vi "dotNETChart_Settings_Default.vi"() -> (2 "Chart Settings clstr":T1={"Enable Mouse Zoom (only works in 2D mode)"=TRUE, "Chart Wall Transparency Level"=37, "Chart Wall Colour"=0, "x axis label"="X axis title", "y axis label"="Y axis title", "Enable3D"=TRUE, "3D Settings"={"Inclination"=20, "LightStyle"=2, "Perspective"=4, "WallWidth"=5, "Rotation"=25}, "BackGradientStyle"=2, "SkinStyle"=1, "Chart Background Gradient Colour"=0, "Chart Border Colour"=0, "Palette"=12, "LegendStyle"=0, "ChartType"=[10, 13], "SeriesDataColour"=[]} {"ChartType" items=["Point", "FastPoint", "Bubble", "Line", "Spline", "StepLine", "FastLine", "Bar", "StackedBar", "StackedBar100", "Column", "StackedColumn", "StackedColumn100", "Area", "SplineArea", "StackedArea", "StackedArea100", "Pie", "Doughnut", "Stock", "Candlestick", "Range", "SplineRange", "RangeBar", "RangeColumn", "Radar", "Polar", "ErrorBar", "BoxPlot", "Renko", "ThreeLineBreak", "Kagi", "PointAndFigure", "Funnel", "Pyramid"]; "LegendStyle" items=["Column", "Row", "Table"]; "Palette" items=["None", "Bright", "Grayscale", "Excel", "Light", "Pastel", "EarthTones", "SemiTransparent", "Berry", "Chocolate", "Fire", "SeaGreen", "BrightPastel"]; "SkinStyle" items=["None", "Emboss", "Raised", "Sunken", "FrameThin1", "FrameThin2", "FrameThin3", "FrameThin4", "FrameThin5", "FrameThin6", "FrameTitle1", "FrameTitle2", "FrameTitle3", "FrameTitle4", "FrameTitle5", "FrameTitle6", "FrameTitle7", "FrameTitle8"]; "BackGradientStyle" items=["None", "LeftRight", "TopBottom", "Center", "DiagonalLeft", "DiagonalRight", "HorizontalCenter", "VerticalCenter"]; "3D Settings"."LightStyle" items=["None", "Simplistic", "Realistic"]})   [LabVIEW 2013, in "dotNETChart XControl.xctl"]
uses:
  dotNETChart XControl.xctl
  typedefs/ChartSettings cluster.ctl
  typedefs/3DSettings.ctl
  typedefs/BackGradientStyle.ctl
  typedefs/SkinStyle.ctl
  typedefs/Palette.ctl
  typedefs/LegendStyle.ctl
  typedefs/ChartType.ctl
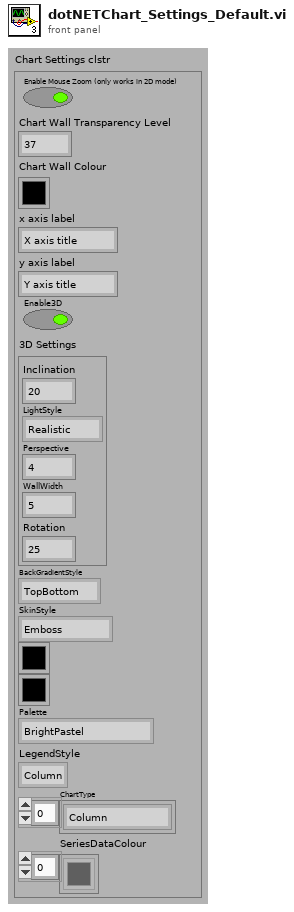
[diagram p1: front panel]
types:
  T1 = typedef "ChartSettings cluster.ctl" = cluster{"Enable Mouse Zoom (only works in 2D mode)":bool, "Chart Wall Transparency Level":i32, "Chart Wall Colour":u32, "x axis label":string, "y axis label":string, "Enable3D":bool, "3D Settings":T2, "BackGradientStyle":T3, "SkinStyle":T4, "Chart Background Gradient Colour":u32, "Chart Border Colour":u32, "Palette":T5, "LegendStyle":T6, "ChartType":T7[], "SeriesDataColour":u32[]}
  T2 = typedef "3DSettings.ctl" = cluster{"Inclination":i32, "LightStyle":i32, "Perspective":i32, "WallWidth":i32, "Rotation":i32}
  T3 = typedef "BackGradientStyle.ctl" = i32
  T4 = typedef "SkinStyle.ctl" = i32
  T5 = typedef "Palette.ctl" = i32
  T6 = typedef "LegendStyle.ctl" = i32
  T7 = typedef "ChartType.ctl" = i32
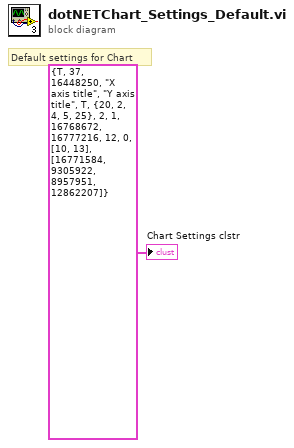
[diagram p0: block diagram]
diagram:
  # "Default settings for Chart"
  "Chart Settings clstr" <- T1 {"Enable Mouse Zoom (only works in 2D mode)"=TRUE, "Chart Wall Transparency Level"=37, "Chart Wall Colour"=16448250, "x axis label"="X axis title", "y axis label"="Y axis title", "Enable3D"=TRUE, "3D Settings"={"Inclination"=20, "LightStyle"=2, "Perspective"=4, "WallWidth"=5, "Rotation"=25}, "BackGradientStyle"=2, "SkinStyle"=1, "Chart Background Gradient Colour"=16768672, "Chart Border Colour"=16777216, "Palette"=12, "LegendStyle"=0, "ChartType"=[10, 13], "SeriesDataColour"=[16771584, 9305922, 8957951, 12862207]} ("Chart Settings clstr")
